vi "Lvlib To Not Parse--constant.vi"() -> (3 "Lvlib Name":string[](array[string]))   [LabVIEW 2021, in "TAF Proj Document Type.lvlib" / "Project Parser.lvlib"]
uses:
  <vilib>/Wovalab/AntiDoc/Document Type/Add-ons/LabVIEW TAF Project/Project Parser/Project Parser.lvlib
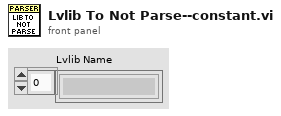
[diagram p1: front panel]
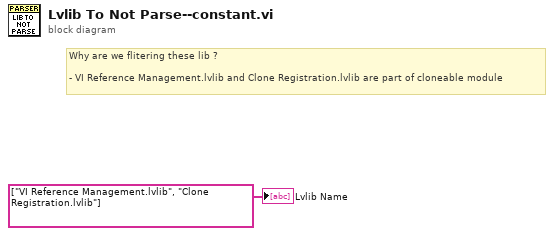
[diagram p0: block diagram]
diagram:
  # "Why are we flitering these lib ?\n\n- VI Reference Management.lvlib and Clone Registration.lvlib are part of cloneable module"
  "Lvlib Name" <- string[] ["VI Reference Management.lvlib", "Clone Registration.lvlib"] ("Lvlib Name")
